vi "Image Normalization.vi"(11 "Input":dbl[][](graph) caption="Image 1") -> (3 "Output":dbl[][](graph) caption="Image 1")   [LabVIEW 2018]
uses:
  <vilib>/Analysis/NI_AALBase.lvlib
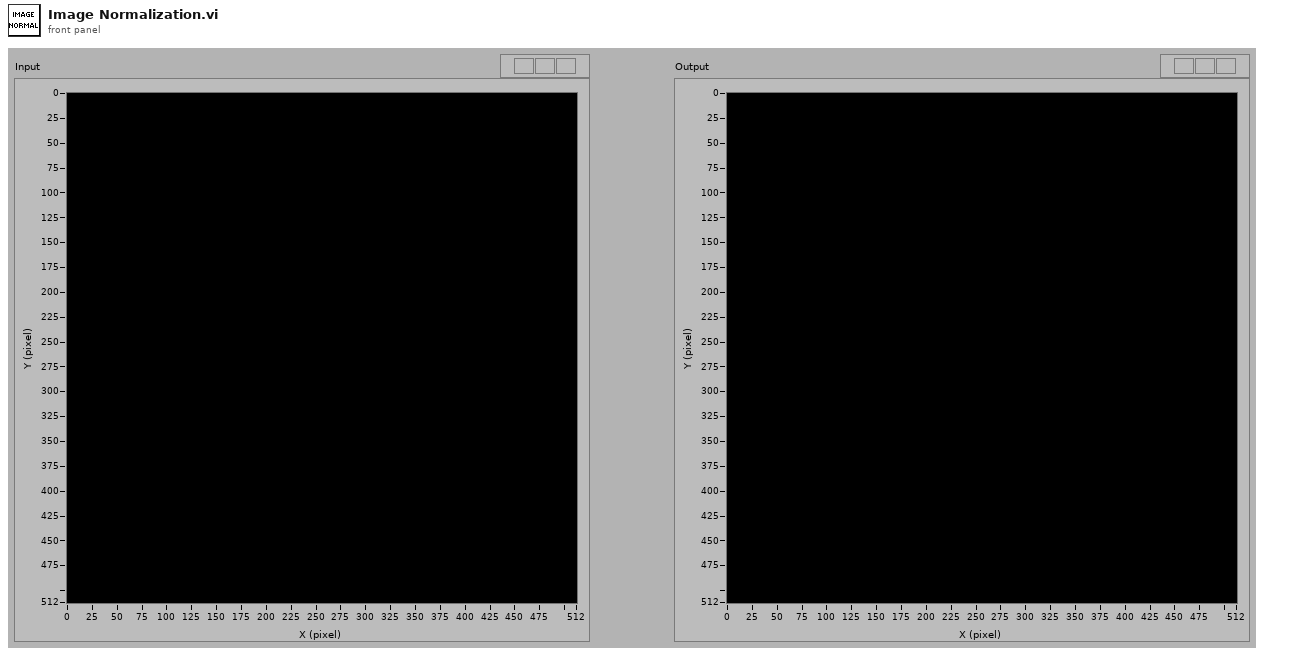
[diagram p1: front panel]
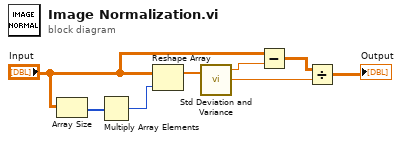
[diagram p0: block diagram]
diagram:
  n1 = Array Size(array="Input") -> (size(s)=w3:i32[])
  n2 = Multiply Array Elements(1:w3) -> (0:w1:i32)
  n3 = Reshape Array("Input", w1) -> (w8:dbl[])
  n4 = call <vilib>:"Std Deviation and Variance.vi"("X"=w8) -> ("mean"=w7:dbl, "standard deviation"=w5:dbl)  [unwired: 1 in, 1 out]
  n5 = Subtract(x="Input", y=w7) -> (x-y=w6:dbl[][])
  n6 = Divide(x=w6, y=w5) -> (x/y=→"Output":dbl[][])
